vi "To HTTP Date String.vi"(11 "Time Stamp":timestamp) -> (3 "HTTP Date":string)   [LabVIEW 2020, in "HTTP Utils.lvlib"]
uses:
  HTTP Utils.lvlib
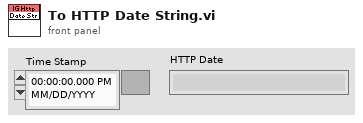
[diagram p1: front panel]
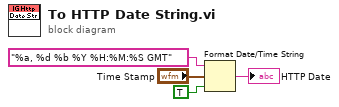
[diagram p0: block diagram]
diagram:
  n1 = Format Date/Time String(time format string (%c)="%a, %d %b %Y %H:%M:%S GMT", seconds (now)="Time Stamp", UTC format=TRUE) -> (date/time string=→"HTTP Date":string)
